vi "Set Name.vi"(8 "error in":errorcluster, 10 "Name":string, 11 "Material-Palette in":refnum<class "Material-Palette.lvclass">) -> (0 "error out":errorcluster, 3 "Material-Palette out":refnum<class "Material-Palette.lvclass">)   [LabVIEW 2021, in "TSC Material Theme.lvlib" / "Material-Palette.lvclass"]
uses:
  Material-Palette.lvclass
  Material-Palette.lvclass/Material-Palette.ctl
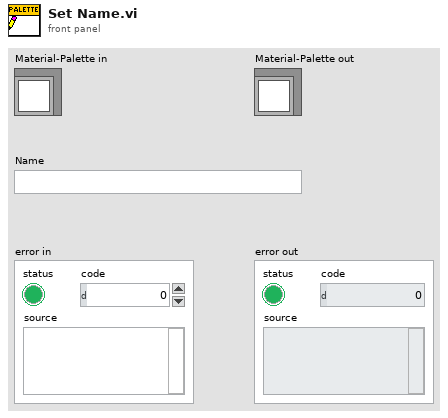
[diagram p1: front panel]
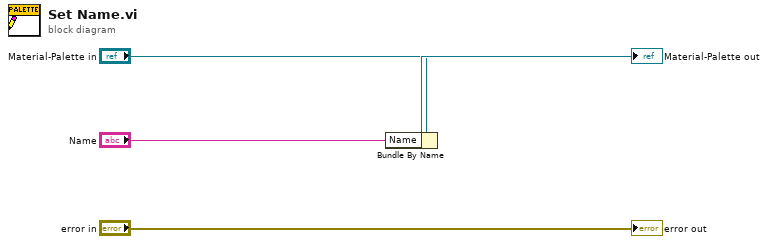
[diagram p0: block diagram]
diagram:
  n1 = Bundle By Name(cluster="Material-Palette in", "Name"="Name") -> (→"Material-Palette out":refnum<class "Material-Palette.lvclass">)
  "error out" <- "error in"
